vi "Analog Data Acquisition and Digital Filtering.vi"() -> ()   [LabVIEW 2018]
uses:
  <vilib>/Utility/error.llb/DialogType.ctl
  <vilib>/DAQmx/read.llb/DAQmx Read (Counter DBL 1Chan 1Samp).vi
  <vilib>/DAQmx/read.llb/DAQmx Read (Analog 1D Wfm NChan NSamp).vi
  <vilib>/DAQmx/create/channels.llb/DAQmx Create Channel (AI-Voltage-Basic).vi
  <vilib>/DAQmx/create/channels.llb/DAQmx Create Channel (CI-Position-Angular Encoder).vi
  <vilib>/DAQmx/configure/timing.llb/DAQmx Timing (Sample Clock).vi
  <vilib>/DAQmx/miscellaneous.llb/DAQmx Fill In Error Info.vi
  <vilib>/measure/macond.llb/IIR Filter for 1 Chan.vi
  <vilib>/Utility/file.llb/Write Delimited Spreadsheet (string).vi
  <vilib>/measure/NI_MAPro.lvlib
panel:
  in  "Number of Samples":dbl=2000.0
  in  "Sample Rate":dbl=1000.0
  in  "Counter":tag="myDAQ1/ctr0"
  in  "maximum value":dbl=5.0
  in  "minimum value":dbl=-5.0
  in  "Analog Physical Channel 1":tag="myDAQ1/ai0"
  in  "Analog Physical Channel 2":tag="myDAQ1/ai1"
  in  "Sensor Sensitivity (mV/g)":i32=289
  in  "decoding type":i32(ring)=10090 items=["X1"=10090, "X2"=10091, "X4"=10092, "Two Pulse Counting"=10313]
  in  "pulses per revolution":u32=480
  in  "file path (dialog if empty)":path=path "C:/Users/Sagar/Desktop/Project1/Test/Integrated programs/testSpreadsheet"
  out "Waveform Graph":waveform(dbl)(graph)
  out "ai1 g Waveform Graph 2":waveform(dbl)(graph)
  out "ai0 g Waveform Graph 2":waveform(dbl)(graph)
  out "ai0 X-axis Waveform Graph":waveform(dbl)[](graph)
  in  "IIR filter specifications":T1={"Topology"=enum."Butterworth", "Type"=enum."Lowpass", "Order"=3, "Lower Fc"=100.0, "Upper Fc"=200.0, "PB Ripple"=1.0, "SB Attenuation"=60.0} {"PB Ripple" format="%0.2f"; "SB Attenuation" format="%0.2f"; "Lower Fc" format="%0.2p"; "Upper Fc" format="%0.2p"}
  out "ai1 Y-axis Waveform Graph":waveform(dbl)[](graph)
  in  "stop":bool
  # "MEE 5318 Project 1\nGroup: 7\nMembers: Sagar Jagtap (903935334)\n                   Arunkumar Ramachandran (903928488)"
  # "Channel Settings"
  # "Timing Settings"
  # "Analog Settings"
  # "Encoder Settings"
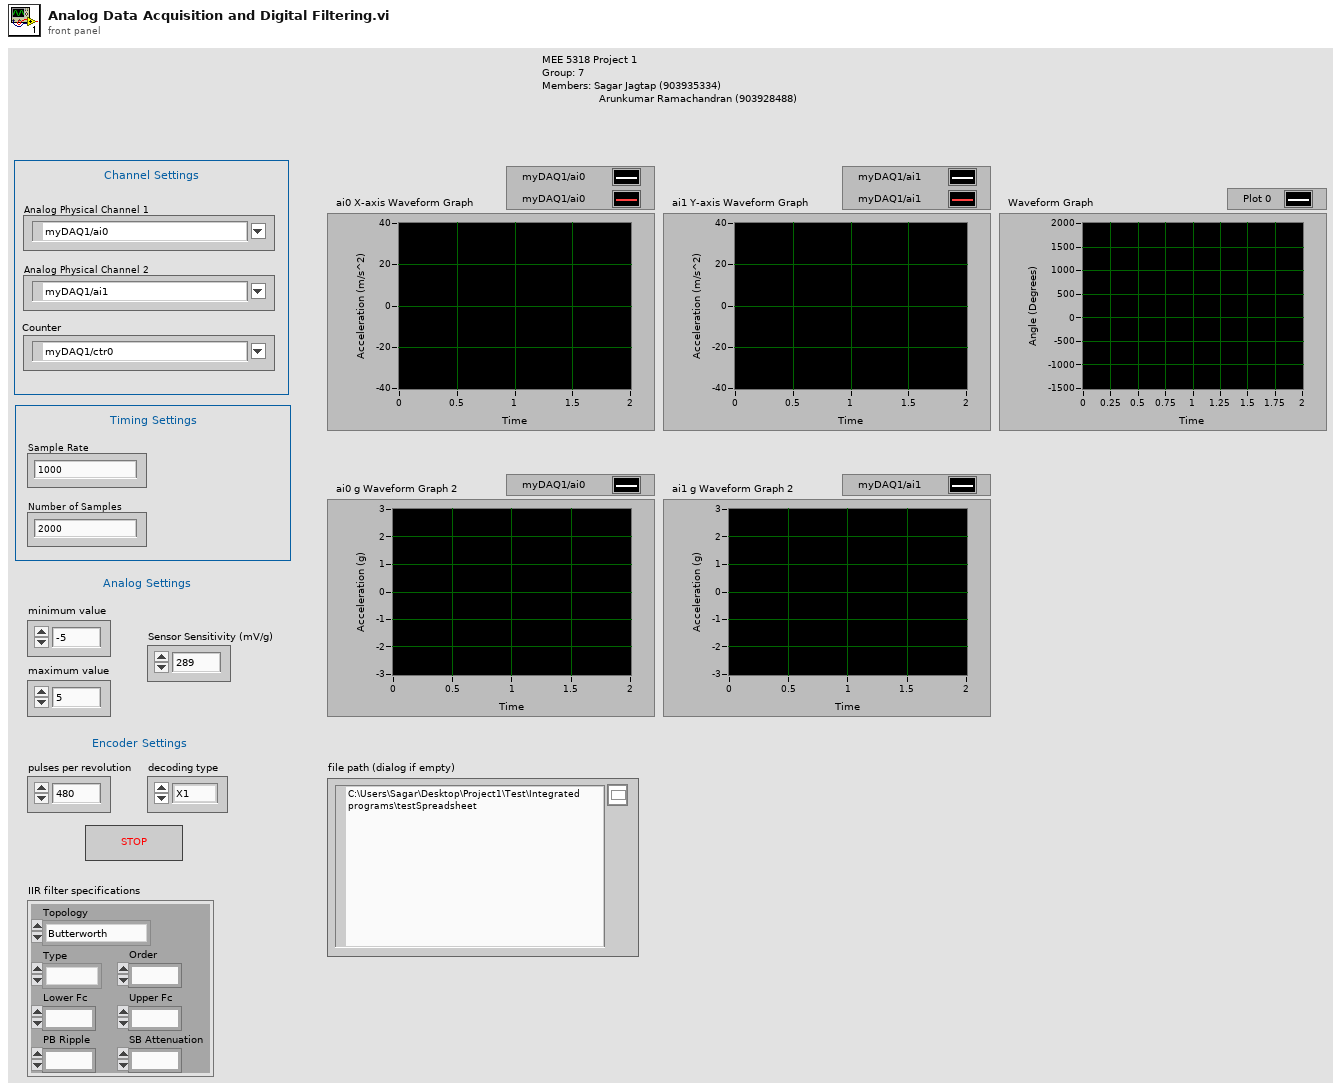
[diagram p1: front panel]
types:
  T1 = cluster{"Topology":enum16{"Off", "Butterworth", "Chebyshev", "Inverse Chebyshev", "Elliptic", "Bessel"}, "Type":enum16{"Lowpass", "Highpass", "Bandpass", "Bandstop"}, "Order":i32, "Lower Fc":dbl, "Upper Fc":dbl, "PB Ripple":dbl, "SB Attenuation":dbl}
  T2 = typedef "DialogType.ctl" = u16
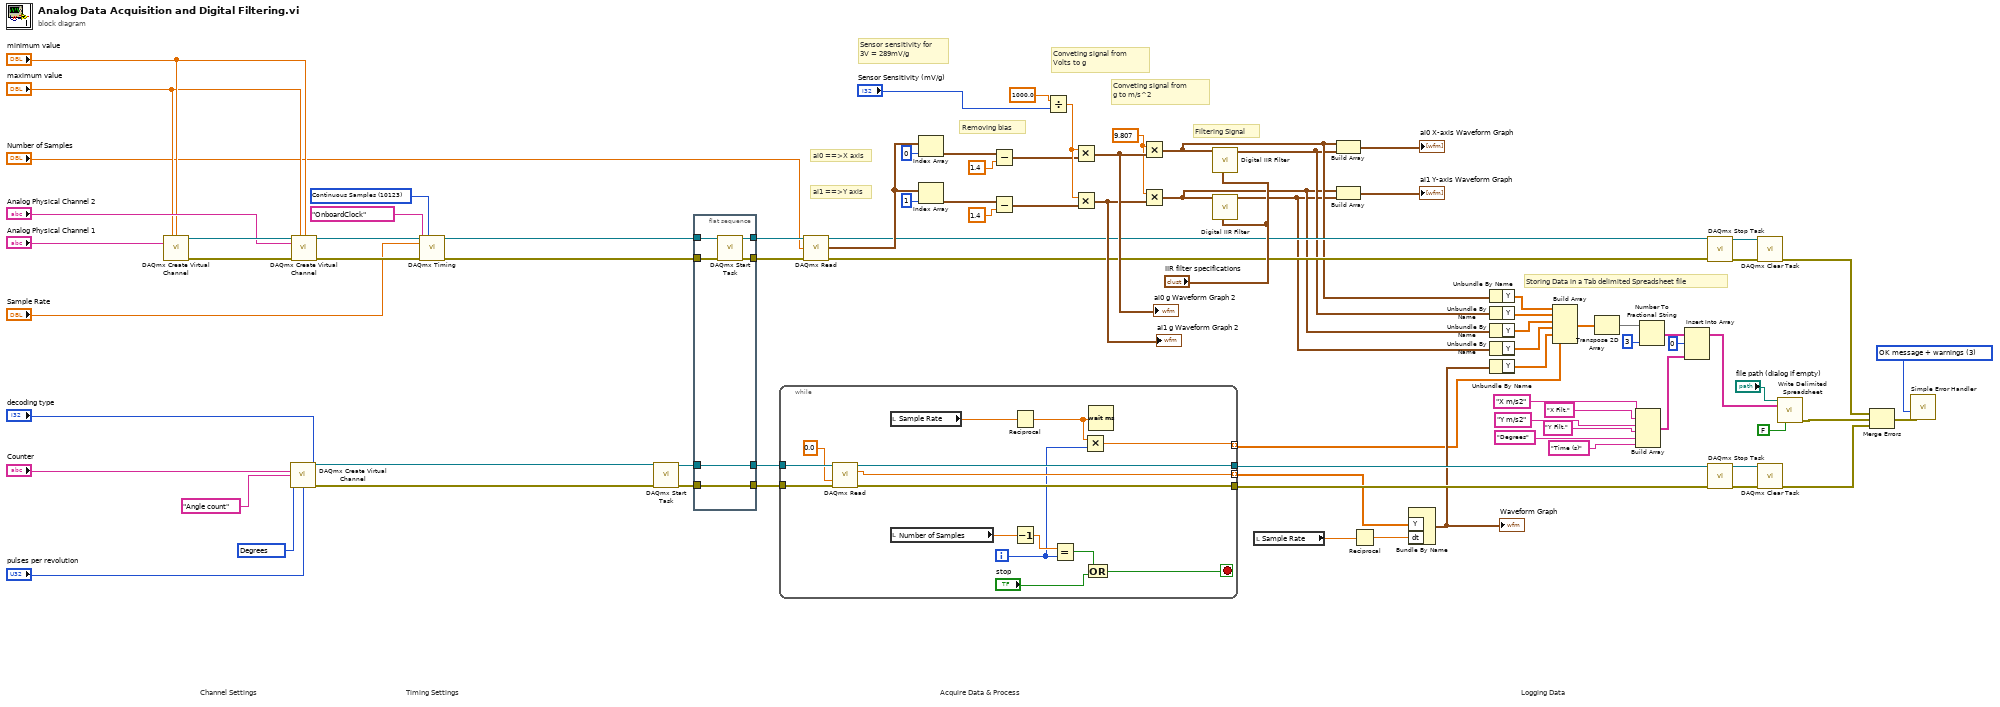
[diagram p0: block diagram]
diagram:
  w48 = T2 3 items=["no dialog", "OK message", "continue or stop message", "OK message + warnings", "continue/stop + warnings"] ("type of dialog (OK msg:1)")
  w47 = 9.807 ("x")
  w73 = 10146 items=["Degrees"=10146, "Radians"=10273, "Ticks"=10304, "From Custom Scale"=10065] ("units")
  w81 = 10123 items=["Finite Samples"=10178, "Continuous Samples"=10123, "Hardware Timed Single Point"=12522] ("sample mode")
  # "Logging Data"
  # "Acquire Data & Process"
  # "Timing Settings"
  # "Channel Settings"
  # "Storing Data in a Tab delimited Spreadsheet file"
  # "ai1 ==>Y axis"
  # "ai0 ==>X axis"
  # "Filtering Signal"
  # "Conveting signal from\ng to m/s^2"
  # "Sensor sensitivity for\n3V = 289mV/g"
  # "Conveting signal from\nVolts to g"
  # "Removing bias"
  n1 = call-poly <vilib>:"DAQmx Create Virtual Channel.vi"("maximum value"="maximum value", "minimum value"="minimum value", "physical channels"="Analog Physical Channel 1") -> ("task out"=w72:refnum<k21>, "error out"=w71:errorcluster)  [unwired: 11 in]
  n2 = call-poly <vilib>:"DAQmx Create Virtual Channel.vi"("counter"="Counter", "decoding type"="decoding type", "name to assign"="Angle count", "units"=w73, "pulses per revolution"="pulses per revolution") -> ("task out"=w80:refnum<k21>, "error out"=w79:errorcluster)  [unwired: 9 in]
  n3 = call-poly <vilib>:"DAQmx Create Virtual Channel.vi"("task in"=w72, "maximum value"="maximum value", "minimum value"="minimum value", "physical channels"="Analog Physical Channel 2", "error in"=w71) -> ("task out"=w70:refnum<k21>, "error out"=w69:errorcluster)  [unwired: 9 in]
  n4 = call-poly <vilib>:"DAQmx Timing.vi"("task/channels in"=w70, "sample mode"=w81, "rate"="Sample Rate", "source"=tag "OnboardClock", "error in"=w69) -> ("task out"=w83:refnum<k21>, "error out"=w82:errorcluster)  [unwired: 9 in]
  n5 = call <vilib>:"DAQmx Start Task.vi"("task/channels in"=w80, "error in"=w79) -> ("task out"=w4:refnum<k21>, "error out"=w2:errorcluster)  [unwired: 12 in]
  n6 = flat-sequence {
    tunnel: w83 -> [w93]
    tunnel: w82 -> [w92]
    tunnel: [w91] -> w54
    tunnel: [w90] -> w53
    tunnel: w4 -> [w89]
    tunnel: [w89] -> w3
    tunnel: w2 -> [w88]
    tunnel: [w88] -> w1
    frame #0 {
      n7 = call <vilib>:"DAQmx Start Task.vi"("task/channels in"=w93, "error in"=w92) -> ("task out"=w91:refnum<k21>, "error out"=w90:errorcluster)  [unwired: 12 in]
    }
  }
  n8 = while {
    tunnel: w3 -> [w108]
    tunnel: w1 -> [w107]
    tunnel: [w106] -> w78
    tunnel: [w105] -> w77
    tunnel: [w101] -> w34 mode=indexing
    tunnel: [w96] -> w22 mode=indexing
    i -> [w97]
    stop <- w103 stop-if-true
    n9 = call-poly <vilib>:"DAQmx Read.vi"("task/channels in"=w108, "timeout"=0.0, "error in"=w107) -> ("task out"=w106:refnum<k21>, "data"=w101:dbl, "error out"=w105:errorcluster)  [unwired: 10 in]
    n10 = local read "Sample Rate"() -> (w95:dbl)
    n11 = local read "Number of Samples"() -> (w98:dbl)
    n12 = Reciprocal(x=w95) -> (1/x=w94:dbl)
    n13 = Decrement(x=w98) -> (x-1=w99:dbl)
    n14 = Equal?(x=w99, y=w97) -> (x = y?=w102:bool)
    n15 = Multiply(x=w94, y=w97) -> (x*y=w96:dbl)
    n16 = Wait (ms)(milliseconds to wait=w94) -> ()  [unwired: 1 out]
    n17 = Compound Arithmetic op=OR(w102, "stop") -> (w103:bool)
  }
  n18 = call-poly <vilib>:"DAQmx Read.vi"("task/channels in"=w54, "number of samples per channel"="Number of Samples", "error in"=w53) -> ("task out"=w51:refnum<k21>, "data"=w61:waveform(dbl)[], "error out"=w50:errorcluster)  [unwired: 10 in]
  n19 = Index Array(array=w61, index=0) -> (element=w62:waveform(dbl))
  n20 = Index Array(array=w61, index=1) -> (element=w64:waveform(dbl))
  n21 = Subtract(x=w62, y=1.4) -> (x-y=w60:waveform(dbl))
  n22 = Subtract(x=w64, y=1.4) -> (x-y=w63:waveform(dbl))
  n23 = Divide(x=1000.0, y="Sensor Sensitivity (mV/g)") -> (x/y=w65:dbl)
  n24 = Multiply(x=w65, y=w60) -> (x*y=w68:waveform(dbl))
  "ai0 g Waveform Graph 2" <- w68
  n25 = Multiply(x=w65, y=w63) -> (x*y=w52:waveform(dbl))
  "ai1 g Waveform Graph 2" <- w52
  n26 = Multiply(x=w47, y=w68) -> (x*y=w44:waveform(dbl))
  n27 = Multiply(x=w47, y=w52) -> (x*y=w42:waveform(dbl))
  n28 = call-poly <vilib>:"Digital IIR Filter.vi"("IIR filter specifications"="IIR filter specifications", "signal in"=w44) -> ("signal out"=w43:waveform(dbl))  [unwired: 7 in, 2 out]
  n29 = call-poly <vilib>:"Digital IIR Filter.vi"("IIR filter specifications"="IIR filter specifications", "signal in"=w42) -> ("signal out"=w41:waveform(dbl))  [unwired: 7 in, 2 out]
  n30 = local read "Sample Rate"() -> (w45:dbl)
  n31 = Build Array(w44, w43) -> (→"ai0 X-axis Waveform Graph":waveform(dbl)[])
  n32 = Build Array(w42, w41) -> (→"ai1 Y-axis Waveform Graph":waveform(dbl)[])
  n33 = Reciprocal(x=w45) -> (1/x=w46:dbl)
  n34 = Bundle By Name("Y"=w34, "dt"=w46) -> (w40:waveform(dbl))  [unwired: 1 in]
  "Waveform Graph" <- w40
  n35 = Unbundle By Name(w44) -> ("Y"=w33:dbl[])
  n36 = Unbundle By Name(w43) -> ("Y"=w39:dbl[])
  n37 = Unbundle By Name(w42) -> ("Y"=w38:dbl[])
  n38 = Unbundle By Name(w41) -> ("Y"=w37:dbl[])
  n39 = Unbundle By Name(w40) -> ("Y"=w36:dbl[])
  n40 = Build Array(w33, w39, w38, w37, w36, w22) -> (w20:dbl[][])
  n41 = Transpose 2D Array(2D array=w20) -> (transposed array=w21:dbl[][])
  n42 = Build Array("X m/s2", "X Filt.", "Y m/s2", "Y Filt.", "Degrees", "Time (s)") -> (w16:string[])
  n43 = Number To Fractional String(number=w21, precision (6)=i16 3) -> (F-format string=w18:string[][])  [unwired: 2 in]
  n44 = Insert Into Array(array=w18, index (row)=0, new element=w16) -> (w15:string[][])  [unwired: 1 in]
  n45 = call <vilib>:"DAQmx Stop Task.vi"("task/channels in"=w51, "error in"=w50) -> ("task out"=w87:refnum<k21>, "error out"=w86:errorcluster)  [unwired: 12 in]
  n46 = call <vilib>:"DAQmx Stop Task.vi"("task/channels in"=w78, "error in"=w77) -> ("task out"=w84:refnum<k21>, "error out"=w85:errorcluster)  [unwired: 12 in]
  n47 = call <vilib>:"DAQmx Clear Task.vi"("task in"=w87, "error in"=w86) -> ("error out"=w75:errorcluster)  [unwired: 13 in]
  n48 = call <vilib>:"DAQmx Clear Task.vi"("task in"=w84, "error in"=w85) -> ("error out"=w29:errorcluster)  [unwired: 13 in]
  n49 = call-poly <vilib>:"Write Delimited Spreadsheet.vi"("file path (dialog if empty)"="file path (dialog if empty)", "2D data"=w15, "transpose? (no:F)"=FALSE) -> ("error out"=w28:errorcluster)  [unwired: 11 in, 1 out]
  n50 = Merge Errors(w75, w28, w29) -> (w76:errorcluster)
  n51 = call <vilib>:"Simple Error Handler.vi"("type of dialog (OK msg:1)"=w48, "error in (no error)"=w76) -> ()  [unwired: 3 in, 5 out]
